vi "zad8.vi"() -> ()   [LabVIEW 2017]
panel:
  in  "stop":bool
  in  "Dodaj":bool
  in  "P³eæ":enum16{"Mê¿czyzna", "Kobieta"}(ring)
  out "Baza Danych":T1
  in  "Aktywny":bool
  in  "Nazwisko":string
  in  "Imie":string
  in  "Wiek":dbl
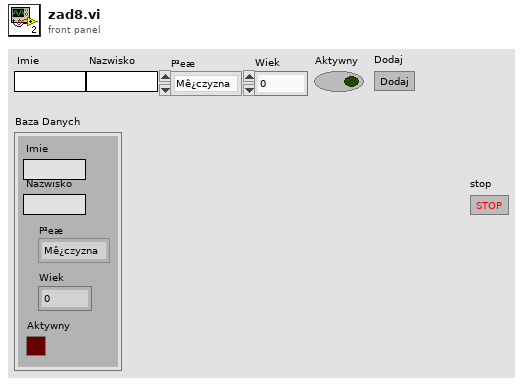
[diagram p1: front panel]
types:
  T1 = cluster{"Imie":string, "Nazwisko":string, "P³eæ":enum16{"Mê¿czyzna", "Kobieta"}, "Wiek":dbl, "Aktywny":bool}
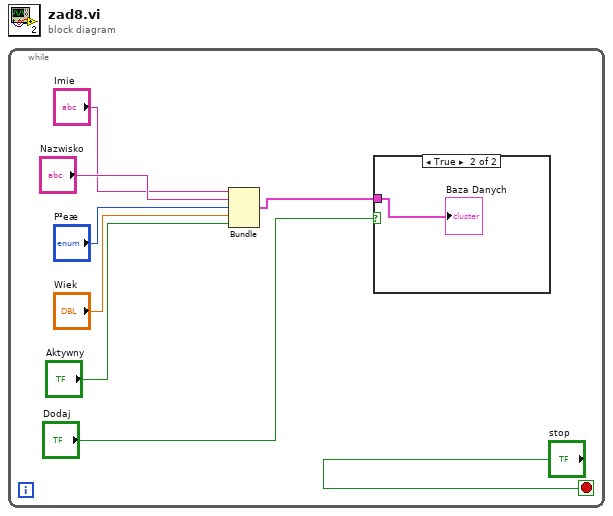
[diagram p0: block diagram]
diagram:
  n1 = while {
    stop <- "stop" stop-if-true
    n2 = Bundle("Imie"="Imie", "Nazwisko"="Nazwisko", "P³eæ"="P³eæ", "Wiek"="Wiek", "Aktywny"="Aktywny") -> (w1:T1)  [unwired: 1 in]
    n3 = case shown="True" "Dodaj" {
      tunnel: w1 -> [_ w9]
      frame False {
      }
      frame True {
        "Baza Danych" <- w9
      }
    }
  }
